vi "ActKeyboardDelete.vi"(8 "Error":errorcluster, 10 "ChatId":i32, 11 "ActKeyboards in":cluster{"ChatId":i32, "Cmd":string}[](array[cluster])) -> (0 "Error":errorcluster, 3 "ActKeyboards out":cluster{"ChatId":i32, "Cmd":string}[](array[cluster]))   [LabVIEW 2015]
uses:
  Telegram/Methods/TypeDefs/CommandList.ctl
panel:
  out "ActKeyboards out":cluster{"Cmd":T1, "ChatId":i32}[](array[cluster])
  in  "ActKeyboards in":cluster{"Cmd":T1, "ChatId":i32}[](array[cluster])
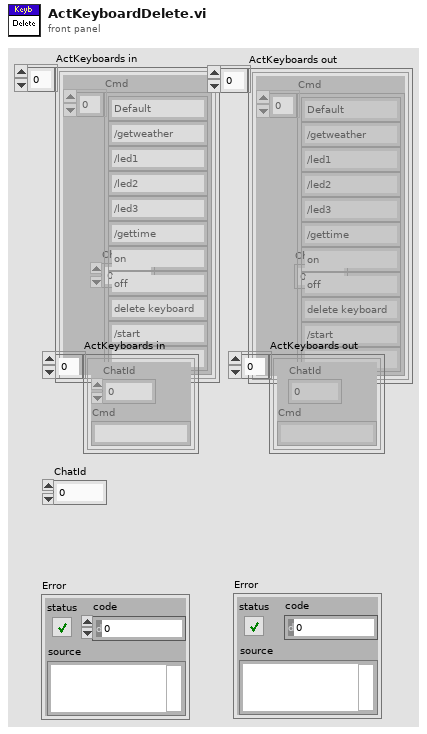
[diagram p1: front panel]
types:
  T1 = typedef "CommandList.ctl" = string[]
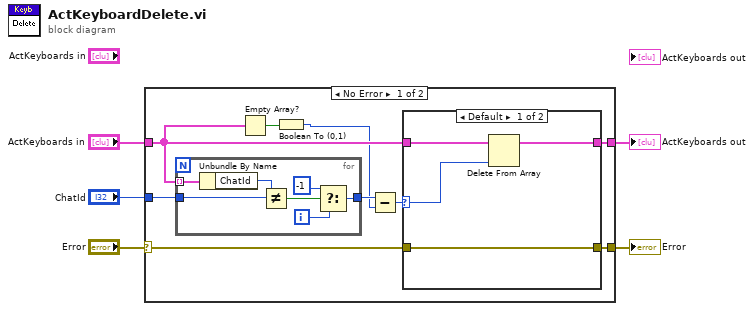
[diagram p0: block diagram]
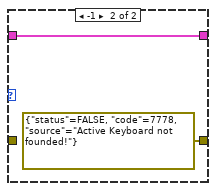
[diagram p2: hidden frame]
diagram:
  n1 = case shown="No Error" "Error" {
    selector: "Error" -> [w12 w29]
    tunnel: [w13 w28] -> w1
    tunnel: "ActKeyboards in" -> [w10 w28]
    tunnel: "ChatId" -> [w14 _]
    tunnel: [w11 w29] -> w3
    frame No Error {
      n2 = for {
        tunnel: w10 -> [w27] mode=indexing
        tunnel: w14 -> [w26]
        tunnel: [w22] -> w8
        i -> [w24]
        n3 = Unbundle By Name(w27) -> ("ChatId"=w21:i32)
        n4 = Not Equal?(x=w21, y=w26) -> (x != y?=w25:bool)
        n5 = Select(t=-1, s=w25, f=w24) -> (s? t:f=w22:i32)
      }
      n6 = Empty Array?(array=w10) -> (empty?=w9:bool)
      n7 = Boolean To (0,1)(Boolean=w9) -> (0, 1=w7:i16)
      n8 = Subtract(x=w8, y=w7) -> (x-y=w6:i32)
      n9 = case shown="Default" w6 {
        selector: w6 -> [w15 _]
        tunnel: [w16 w20] -> w13
        tunnel: w10 -> [w17 w20]
        tunnel: w12 -> [w18 _]
        tunnel: [w18 errorcluster {"status"=FALSE, "code"=7778, "source"="Active Keyboard not founded!"} ("t")] -> w11
        frame Default {
          n10 = Delete From Array(array=w17, index=w15) -> (array with subset deleted=w16:cluster{"ChatId":i32, "Cmd":string}[])  [unwired: 1 in, 1 out]
        }
        frame -1 {
        }
      }
    }
    frame Error {
    }
  }
  "Error" <- w3
  "ActKeyboards out" <- w1
